vi "Real Robot Car.vi"() -> ()   [LabVIEW 2016]
panel:
  out "Boolean 4":bool
  out "Boolean 3":bool
  out "Boolean":bool
  out "Boolean 2":bool
  out "Boolean":bool
  out "Boolean":bool
  in  "Turn Left Array 2":bool[](array[boolean]) caption="Turn Left"
  in  "Forward Array 2":bool[](array[boolean]) caption="Forward"
  in  "Turn Right Array 2":bool[](array[boolean]) caption="Turn Right"
  in  "Stop Array 2":bool[](array[boolean]) caption="Stop"
  out "Right PR Black":bool
  out "Mid PR Black":bool
  out "Left PR Black":bool
  out "Right PR Voltage 3":dynamicdata(graph)
  out "Right PR (volts) 3":dbl
  out "Mid PR Voltage 2":dynamicdata(graph)
  out "Mid PR (volts) 2":dbl
  out "Left PR Voltage":dynamicdata(graph)
  out "Right IR Voltage":dynamicdata(graph)
  out "Mid IR Voltage":dynamicdata(graph)
  out "Left IR Voltage":dynamicdata(graph)
  out "Left PR (volts)":dbl
  out "Voltage 3":dbl
  out "Right IR":bool
  out "Voltage 2":dbl
  out "Middle IR":bool
  out "Left IR":bool
  out "Voltage":dbl
  in  "stop":bool
  in  "Backward Array":bool[](array[boolean]) caption="Backward"
  # "NOTE: This is the final VI for your project. \nWhat you need to do is complete this template by\nadding the boolean (digital) logic on the back panel.\n(See block diagram)"
  # "Indicates if comparison on block diagram is true."
  # "Set your array values. For a value of 1, \nclick on the dot and make it turn black.\nFor a value of zero, leave the dot light gray"
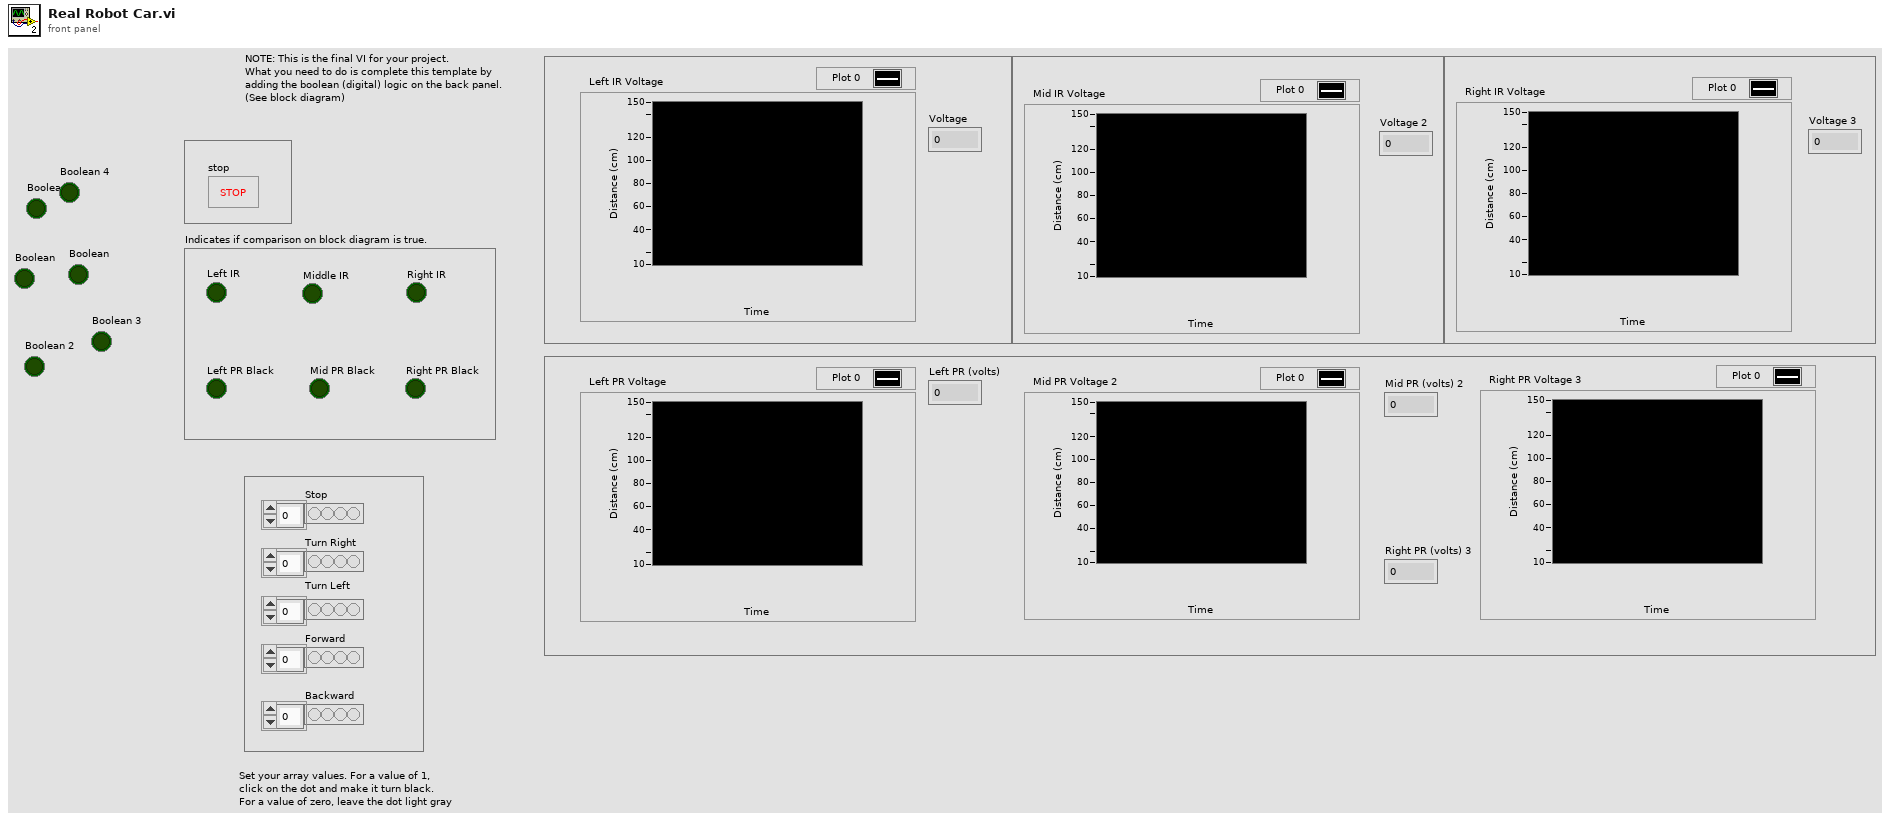
[diagram p1: front panel]
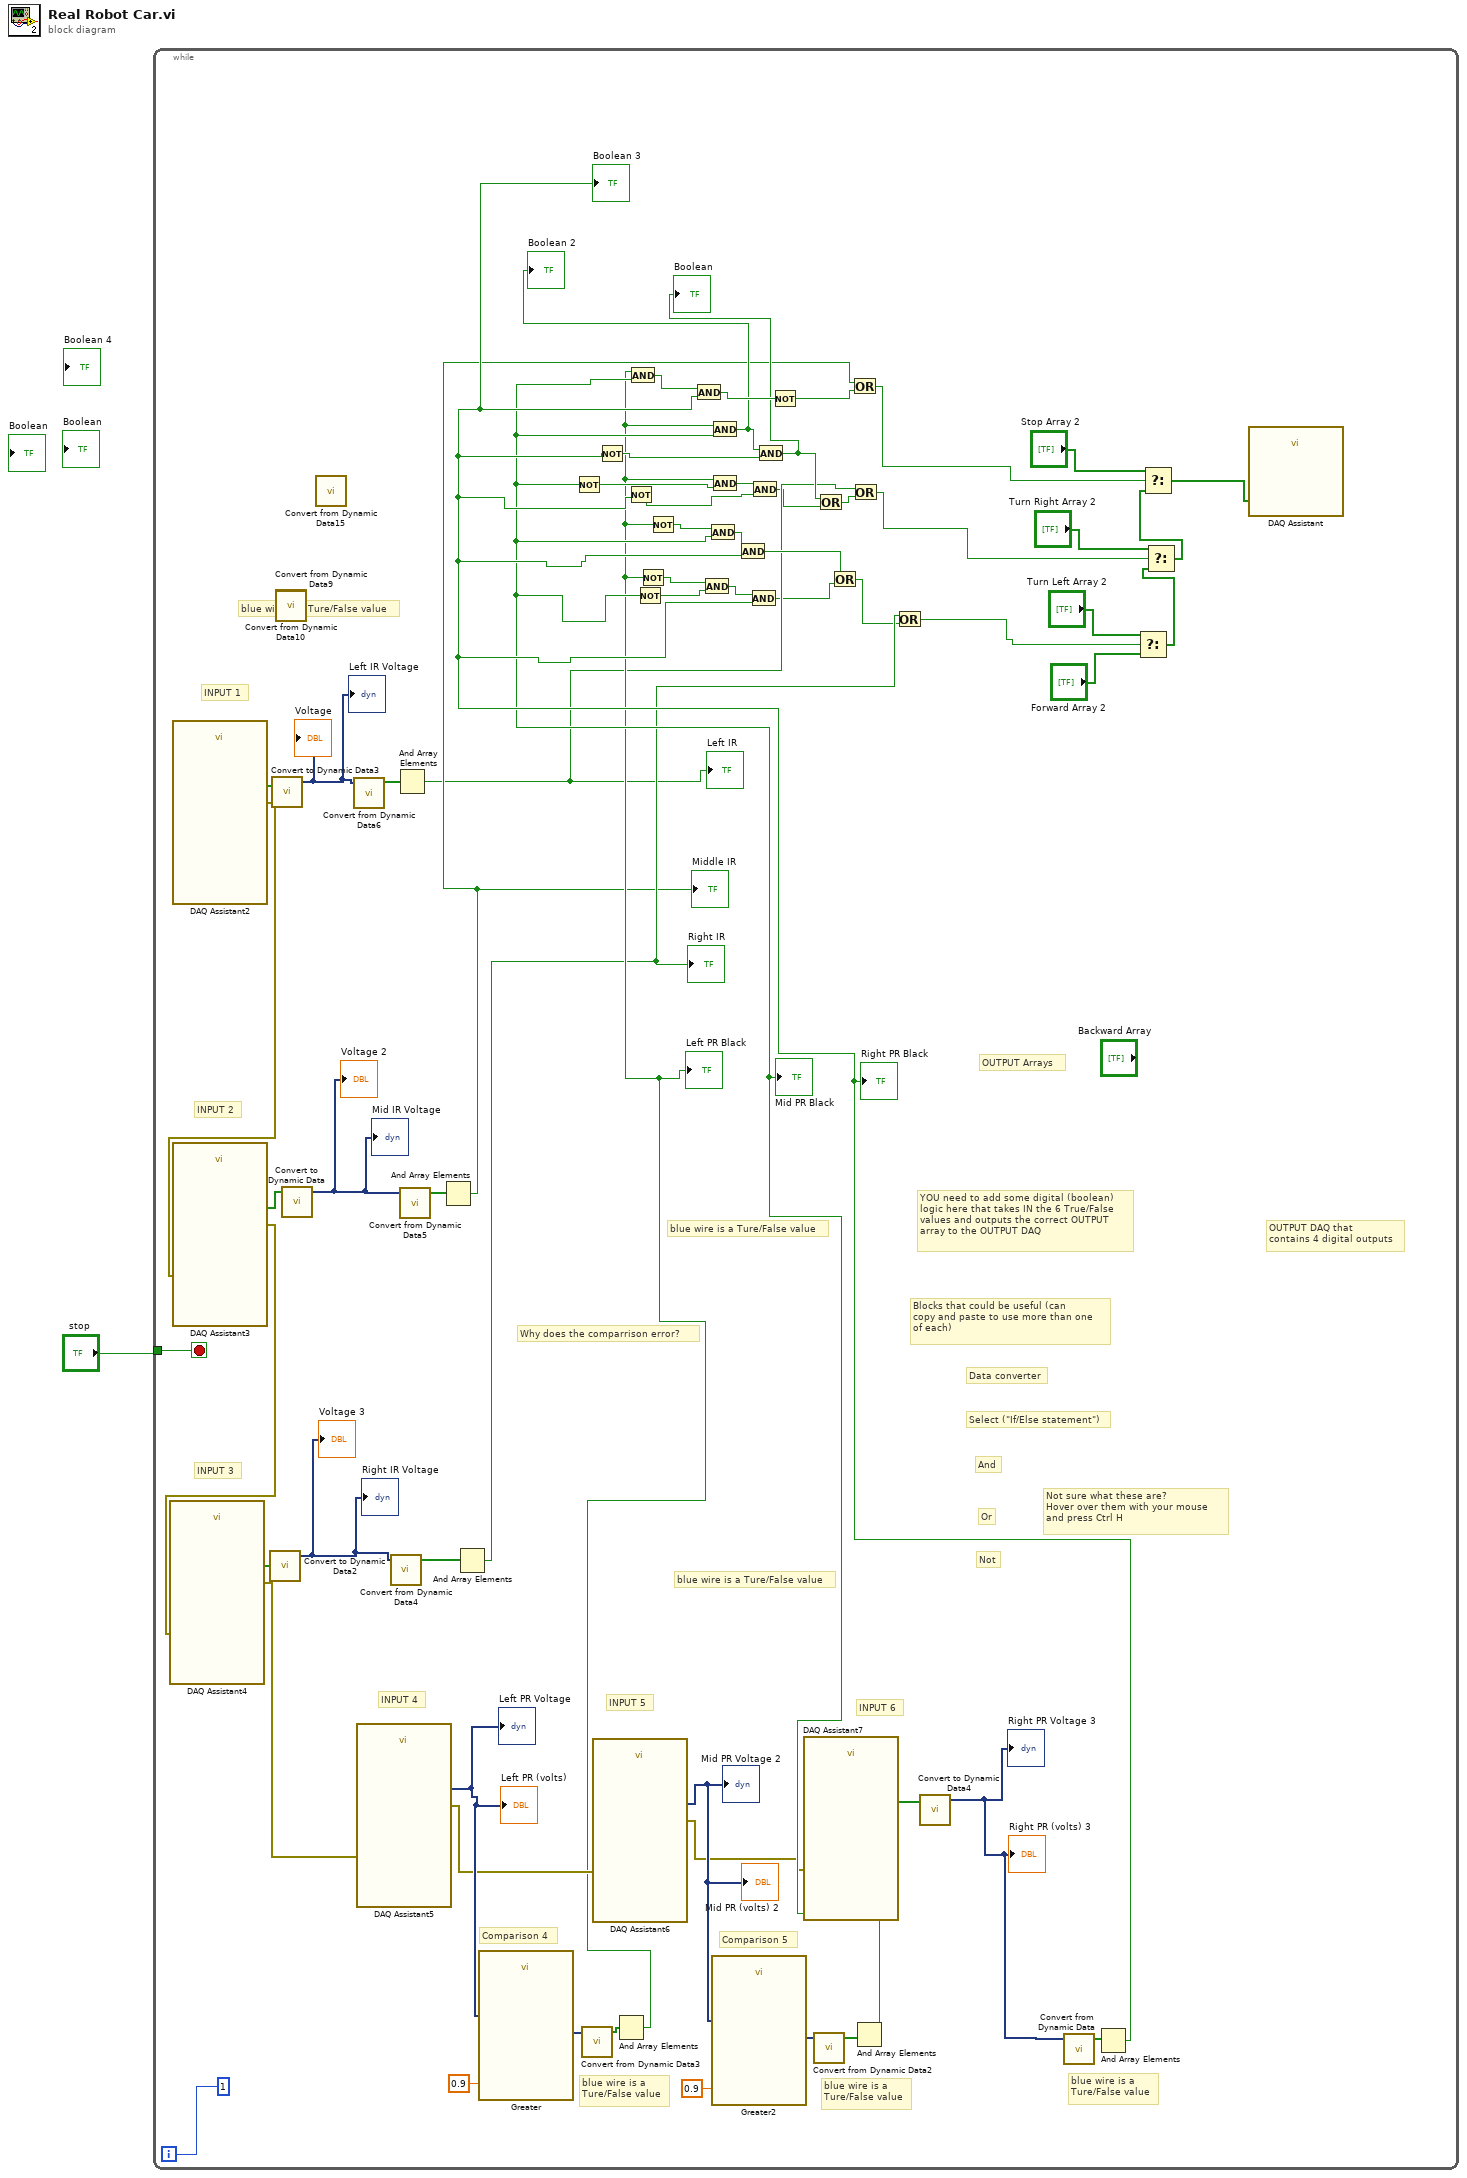
[diagram p0: block diagram]
diagram:
  n1 = while {
    tunnel: "stop" -> [w63]
    i -> [1]
    stop <- w63 stop-if-true
    # "Why does the comparrison error?"
    # "Not sure what these are? \nHover over them with your mouse\nand press Ctrl H"
    # "Not"
    # "Or"
    # "And"
    # "Select (\"If/Else statement\")"
    # "Data converter"
    # "Blocks that could be useful (can \ncopy and paste to use more than one\nof each)"
    # "YOU need to add some digital (boolean)\nlogic here that takes IN the 6 True/False \nvalues and outputs the correct OUTPUT \narray to the OUTPUT DAQ"
    # "blue wire is a \nTure/False value"
    # "blue wire is a\nTure/False value"
    # "blue wire is a \nTure/False value"
    # "blue wire is a Ture/False value"
    # "blue wire is a Ture/False value"
    # "blue wire is a Ture/False value"
    # "OUTPUT DAQ that\ncontains 4 digital outputs"
    # "OUTPUT Arrays"
    # "INPUT 6"
    # "Comparison 5"
    # "INPUT 5"
    # "Comparison 4"
    # "INPUT 4"
    # "INPUT 3"
    # "INPUT 2"
    # "INPUT 1"
    n2 = call "DAQ Assistant2"() -> ("data"=w60:bool[], "error out"=w59:errorcluster)  [unwired: 17 in, 1 out]
    n3 = call "DAQ Assistant3"("error in"=w59) -> ("data"=w56:bool[], "error out"=w58:errorcluster)  [unwired: 16 in, 1 out]
    n4 = call "DAQ Assistant4"("error in"=w58) -> ("data"=w55:bool[], "error out"=w57:errorcluster)  [unwired: 16 in, 1 out]
    n5 = call "Convert to Dynamic Data2"("Array"=w55) -> ("Dynamic Data Type"=w22:dynamicdata)  [unwired: 3 in]
    "Voltage 3" <- w22
    "Right IR Voltage" <- w22
    n6 = call "Convert to Dynamic Data3"("Array"=w60) -> ("Dynamic Data Type"=w16:dynamicdata)  [unwired: 3 in]
    "Voltage" <- w16
    "Left IR Voltage" <- w16
    n7 = call "Convert from Dynamic Data10"() -> ()  [unwired: 4 in, 1 out]
    n8 = call "Convert from Dynamic Data9"() -> ()  [unwired: 4 in, 1 out]
    n9 = call "Convert to Dynamic Data"("Array"=w56) -> ("Dynamic Data Type"=w19:dynamicdata)  [unwired: 3 in]
    "Voltage 2" <- w19
    "Mid IR Voltage" <- w19
    n10 = call "Convert from Dynamic Data15"() -> ()  [unwired: 4 in, 1 out]
    n11 = call "Convert from Dynamic Data6"("Dynamic Data Type"=w16) -> ("Array"=w15:bool[])  [unwired: 3 in]
    n12 = call "DAQ Assistant5"("error in"=w57) -> ("data"=w54:dynamicdata, "error out"=w53:errorcluster)  [unwired: 16 in, 1 out]
    "Left PR (volts)" <- w54
    "Left PR Voltage" <- w54
    n13 = call "Convert from Dynamic Data4"("Dynamic Data Type"=w22) -> ("Array"=w21:bool[])  [unwired: 3 in]
    n14 = And Array Elements(Boolean array=w15) -> (logical AND=w14:bool)
    "Left IR" <- w14
    n15 = call "Convert from Dynamic Data5"("Dynamic Data Type"=w19) -> ("Array"=w18:bool[])  [unwired: 3 in]
    n16 = And Array Elements(Boolean array=w18) -> (logical AND=w17:bool)
    "Middle IR" <- w17
    n17 = And Array Elements(Boolean array=w21) -> (logical AND=w20:bool)
    "Right IR" <- w20
    n18 = call "Greater"("Constant Value to Compare Against"=0.9, "Operand 1"=w54) -> ("Result"=w25:dynamicdata)  [unwired: 8 in, 1 out]
    n19 = call "Convert from Dynamic Data3"("Dynamic Data Type"=w25) -> ("Array"=w24:bool[])  [unwired: 3 in]
    n20 = call "DAQ Assistant6"("error in"=w53) -> ("data"=w52:dynamicdata, "error out"=w5:errorcluster)  [unwired: 16 in, 1 out]
    "Mid PR (volts) 2" <- w52
    "Mid PR Voltage 2" <- w52
    n21 = And Array Elements(Boolean array=w24) -> (logical AND=w23:bool)
    "Left PR Black" <- w23
    n22 = Not(x=w23) -> (.not. x?=w39:bool)
    n23 = Not(x=w23) -> (.not. x?=w37:bool)
    n24 = call "Greater2"("Constant Value to Compare Against"=0.9, "Operand 1"=w52) -> ("Result"=w28:dynamicdata)  [unwired: 8 in, 1 out]
    n25 = call "DAQ Assistant7"("error in"=w5) -> ("data"=w4:bool[])  [unwired: 16 in, 2 out]
    n26 = call "Convert from Dynamic Data2"("Dynamic Data Type"=w28) -> ("Array"=w27:bool[])  [unwired: 3 in]
    n27 = And Array Elements(Boolean array=w27) -> (logical AND=w26:bool)
    "Mid PR Black" <- w26
    n28 = Not(x=w26) -> (.not. x?=w35:bool)
    n29 = And(x=w23, y=w26) -> (x .and. y?=w51:bool)
    n30 = Not(x=w26) -> (.not. x?=w38:bool)
    n31 = And(x=w39, y=w38) -> (x .and. y?=w42:bool)
    n32 = And(x=w37, y=w26) -> (x .and. y?=w43:bool)
    n33 = And(x=w23, y=w26) -> (x .and. y?=w33:bool)
    "Boolean 2" <- w33
    n34 = And(x=w23, y=w35) -> (x .and. y?=w44:bool)
    n35 = call "Convert to Dynamic Data4"("Array"=w4) -> ("Dynamic Data Type"=w3:dynamicdata)  [unwired: 3 in]
    "Right PR (volts) 3" <- w3
    "Right PR Voltage 3" <- w3
    n36 = call "Convert from Dynamic Data"("Dynamic Data Type"=w3) -> ("Array"=w30:bool[])  [unwired: 3 in]
    n37 = And Array Elements(Boolean array=w30) -> (logical AND=w29:bool)
    "Right PR Black" <- w29
    "Boolean 3" <- w29
    n38 = Not(x=w29) -> (.not. x?=w31:bool)
    n39 = Not(x=w29) -> (.not. x?=w36:bool)
    n40 = And(x=w51, y=w29) -> (x .and. y?=w41:bool)
    n41 = And(x=w43, y=w29) -> (x .and. y?=w40:bool)
    n42 = And(x=w42, y=w29) -> (x .and. y?=w13:bool)
    n43 = And(x=w44, y=w36) -> (x .and. y?=w11:bool)
    n44 = And(x=w33, y=w31) -> (x .and. y?=w32:bool)
    "Boolean" <- w32
    n45 = Not(x=w41) -> (.not. x?=w9:bool)
    n46 = Or(x=w32, y=w11) -> (x .or. y?=w10:bool)
    n47 = Or(x=w40, y=w13) -> (x .or. y?=w12:bool)
    n48 = Or(x=w17, y=w9) -> (x .or. y?=w7:bool)
    n49 = Or(x=w14, y=w10) -> (x .or. y?=w8:bool)
    n50 = Or(x=w20, y=w12) -> (x .or. y?=w6:bool)
    n51 = Select(t="Turn Left Array 2", s=w6, f="Forward Array 2") -> (s? t:f=w47:bool[])
    n52 = Select(t="Turn Right Array 2", s=w8, f=w47) -> (s? t:f=w46:bool[])
    n53 = Select(t="Stop Array 2", s=w7, f=w46) -> (s? t:f=w34:bool[])
    n54 = call "DAQ Assistant"("data"=w34) -> ()  [unwired: 17 in, 2 out]
  }
